vi "Lab Panel V6.00.vi"() -> ()   [LabVIEW 2017] (continued)
                          frame "CHART TEST", Default {
                          }
                          frame "CYCLE TEST" {
                          }
                          frame "T-RISE TEST" {
                          }
                        }
                        n877 = local read "TDMS LAB03-2"() -> (w1509:refnum<k34>)
                        n878 = Build Array("STOPPED") -> (w1506:string[])
                        n879 = Build Array(w1501) -> (w1500:dbl[])
                        n880 = TDMS Write(0:w1509, 5:"TEST RESULT", 7:w1506, 9:w1500) -> (4:w1498:refnum<k34>, 15:w1499:errorcluster)  [unwired: 2 in, 2 out]
                        n881 = TDMS Close(8:w1499, 11:w1498) -> (0:w1497:errorcluster)  [unwired: 1 out]
                      }
                      frame #1 {
                        n882 = local read "DISP LAB03-2"() -> (w1516:T4)
                        n883 = stacked-sequence {
                          tunnel: "LAB03-2" -> [w1518 w1520]
                          frame #0 {
                            n884 = call "sub vi - defrag tdms v1.vi"("panel id"=w1518) -> ("error out"=w1517:errorcluster)  [unwired: 10 in]
                            n885 = local write "data file error"(w1517) -> ()
                          }
                          frame #1 {
                            n886 = call "Save data file (stop) v3.vi"("panel id"=w1520) -> ("network file save error"=w1519:errorcluster)  [unwired: 9 in, 1 out]
                            n887 = local write "RESULT LAB03-2"(FALSE) -> ()
                            n888 = local write "data file error"(w1519) -> ()
                          }
                        }
                        n889 = Bundle(cluster=w1516, "STATUS"="STOP") -> (w1514:T4)  [unwired: 2 in]
                        n890 = local write "DISP LAB03-2"(w1514) -> ()
                      }
                    }
                  }
                  frame True {
                    n891 = local read "SIG LAB03-2"() -> (w1523:T2)
                    n892 = stacked-sequence {
                      seq-local: [w1534 _] -> [_ w1538]
                      tunnel: w1532 -> [_ w1548]
                      tunnel: w1531 -> [_ w1547]
                      tunnel: w1530 -> [_ w1546]
                      tunnel: w1529 -> [_ w1545]
                      tunnel: w1528 -> [_ w1544]
                      tunnel: [_ w1543] -> w1527
                      tunnel: w1526 -> [_ w1542]
                      tunnel: w1525 -> [_ w1541]
                      tunnel: w1524 -> [_ w1540]
                      tunnel: w1523 -> [w1533 w1539]
                      tunnel: w1522 -> [_ w1537]
                      frame #0 {
                        n893 = Unbundle(w1533) -> ("AMPS"=w1536:dbl)  [unwired: 4 out]
                        n894 = call "Check For Amps on v1.vi"("ID"="LAB03-2", "amps"=w1536) -> ("amps"=w1534:bool)  [unwired: 9 in]
                      }
                      frame #1 {
                        n895 = case shown="True" w1538 {
                          tunnel: w1548 -> [_ w1561]
                          tunnel: w1547 -> [_ w1560]
                          tunnel: w1546 -> [_ w1559]
                          tunnel: w1545 -> [_ w1558]
                          tunnel: w1544 -> [_ w1557]
                          tunnel: [errorcluster {"status"=FALSE, "code"=0, "source"=""} ("error out") w1556] -> w1543
                          tunnel: w1542 -> [_ w1555]
                          tunnel: w1541 -> [_ w1554]
                          tunnel: w1540 -> [_ w1553]
                          tunnel: w1539 -> [_ w1552]
                          tunnel: w1537 -> [_ w1551]
                          frame False {
                            w1549 = FALSE
                            n896 = local write "RUN LAB03-2"(w1549) -> ()
                            n897 = local write "run lab03-2"(w1549) -> ()
                          }
                          frame True {
                            n898 = stacked-sequence {
                              seq-local: [w1562 _ _ _ _] -> [_ w1586 _ _ _]
                              tunnel: w1561 -> [w1567 _ _ _ _]
                              tunnel: w1560 -> [w1564 _ _ _ _]
                              tunnel: w1559 -> [w1577 _ _ _ _]
                              tunnel: w1558 -> [w1570 _ _ _ _]
                              tunnel: w1557 -> [w1565 _ _ _ _]
                              tunnel: [_ w1581 _ _ _] -> w1556
                              tunnel: w1555 -> [_ _ _ w1607 _]
                              tunnel: w1554 -> [_ _ _ w1606 _]
                              tunnel: w1553 -> [_ _ _ w1605 _]
                              tunnel: w1552 -> [_ _ _ _ _]
                              tunnel: w1551 -> [_ _ _ _ w1621]
                              frame #0 {
                                w1563 = "\\"
                                n899 = local read "SET LAB03-2"() -> (w1572:T5)
                                n900 = case shown="\"T-RISE TEST\"" w1577 {
                                tunnel: ["L03-2-CHART TEST-" "L03-2-CYCLE TEST-" "L03-2-T-RISE TEST-"] -> w1573
                                frame "CHART TEST", Default {
                                }
                                frame "CYCLE TEST" {
                                }
                                frame "T-RISE TEST" {
                                }
                                }
                                n901 = Unbundle(w1572) -> ("DESCRIPTION"=w1571:string)  [unwired: 4 out]
                                n902 = Concatenate Strings(w1567, "\\", w1565, w1563, w1564, w1563) -> (w1574:string)
                                n903 = String To Path(string=w1574) -> (path=w1576:path)
                                n904 = Concatenate Strings(w1574, w1573, w1571, "-", w1570, ".tdms") -> (w1562:string)
                                n905 = Create Folder(path (use dialog)=w1576) -> (error out=w1575:errorcluster)  [unwired: 2 in, 2 out]
                                n906 = global write "Global 1.vi" "LAB03-2 FILE"(w1562) -> ()
                                n907 = call <vilib>:"Clear Errors.vi"("error in (no error)"=w1575) -> ()  [unwired: 5 in, 2 out]
                              }
                              frame #1 {
                                (unwired) FALSE
                                n908 = String To Path(string=w1586) -> (path=w1582:path)
                                n909 = TDMS Open(6:FALSE, 10:T23."create or replace" ("operation (0:open)"), 11:w1582) -> (0:w1581:errorcluster, 3:→"TDMS LAB03-2":refnum<k34>)  [unwired: 4 in]
                              }
                              frame #2 {
                                n910 = local read "SET LAB03-2"() -> (w1592:T5)
                                n911 = local read "TDMS LAB03-2"() -> (w1603:refnum<k34>)
                                n912 = Build Array("Testers Name", "Description", "Set Test Cycles", "T-Rise minutes", "T-Rise Deg C") -> (w1593:string[])
                                n913 = Unbundle(w1592) -> ("NAME"=w1591:string, "DESCRIPTION"=w1590:string, "CYCLES"=w1589:dbl, "T-RISE mins"=w1588:dbl, "T-RISE deg C"=w1587:dbl)
                                n914 = Number To Decimal String(number=w1589) -> (decimal integer string=w1602:string)  [unwired: 1 in]
                                n915 = Number To Decimal String(number=w1588) -> (decimal integer string=w1601:string)  [unwired: 1 in]
                                n916 = Number To Decimal String(number=w1587) -> (decimal integer string=w1600:string)  [unwired: 1 in]
                                n917 = Build Array(w1591, w1590, w1602, w1601, w1600) -> (w1599:string[])
                                n918 = TDMS Set Properties(5:w1599, 7:w1593, 11:w1603) -> ()  [unwired: 3 in, 4 out]
                              }
                              frame #3 {
                                n919 = local read "DISP LAB03-2"() -> (w1608:T4)
                                n920 = Concatenate Strings("LAB03-2  ", w1607) -> (w1609:string)
                                n921 = Two Button Dialog(message=w1609, 1:w1605, 2:w1606) -> (T button?=w1611:bool)
                                n922 = case shown="True" w1611 {
                                tunnel: w1608 -> [w1618 w1619]
                                tunnel: [w1618 w1619] -> w1615
                                tunnel: [w1617 w1620] -> w1614
                                tunnel: [w1616 w1620] -> w1613
                                frame False {
                                n923 = Unbundle(w1618) -> ("CYCLE"=w1617:dbl, "MINS"=w1616:dbl)  [unwired: 1 out]
                                }
                                frame True {
                                w1620 = 0.0
                                }
                                }
                                n924 = Bundle(cluster=w1615, "CYCLE"=w1614, "MINS"=w1613, "STATUS"="RUN") -> (w1604:T4)
                                n925 = local write "DISP LAB03-2"(w1604) -> ()
                              }
                              frame #4 {
                                n926 = local read "TEMP START LAB03-2"() -> (w1623:cluster{"TL":dbl, "TN":dbl})
                                n927 = Bundle(cluster=w1623, "TL"=w1621, "TN"=w1621) -> (w1622:cluster{"TL":dbl, "TN":dbl})
                                n928 = local write "TEMP START LAB03-2"(w1622) -> ()
                              }
                            }
                          }
                        }
                      }
                    }
                  }
                }
              }
              event "RUN LAB04-1": Value Change {
                n929 = event-data() -> ("NewVal"=w1628:bool)  [unwired: 1 in, 5 out]
                n930 = local write "run lab04-1"(w1628) -> ()
                n931 = case shown="True" w1628 {
                  tunnel: w1634 -> [_ w1672]
                  tunnel: w1633 -> [_ w1671]
                  tunnel: w1631 -> [w1636 w1670]
                  tunnel: w1632 -> [_ w1669]
                  tunnel: w1630 -> [_ w1668]
                  tunnel: [w1635 w1667] -> w1629
                  tunnel: w1627 -> [_ w1666]
                  tunnel: w1626 -> [_ w1665]
                  tunnel: w1625 -> [_ w1664]
                  tunnel: w1624 -> [_ w1662]
                  frame False {
                    # "stop test"
                    n932 = stacked-sequence {
                      tunnel: w1636 -> [w1645 _]
                      tunnel: [w1637 _] -> w1635
                      frame #0 {
                        n933 = local read "DISP LAB04-1"() -> (w1644:T4)
                        n934 = Unbundle(w1644) -> ("CYCLE"=w1642:dbl, "MINS"=w1643:dbl)  [unwired: 1 out]
                        n935 = case shown="\"CYCLE TEST\"" w1645 {
                          tunnel: w1643 -> [_ _ w1652]
                          tunnel: w1642 -> [w1650 w1651 _]
                          tunnel: [w1650 w1651 w1652] -> w1641
                          frame "CHART TEST", Default {
                          }
                          frame "CYCLE TEST" {
                          }
                          frame "T-RISE TEST" {
                          }
                        }
                        n936 = local read "TDMS LAB04-1"() -> (w1649:refnum<k34>)
                        n937 = Build Array("STOPPED") -> (w1646:string[])
                        n938 = Build Array(w1641) -> (w1640:dbl[])
                        n939 = TDMS Write(0:w1649, 5:"TEST RESULT", 7:w1646, 9:w1640) -> (4:w1638:refnum<k34>, 15:w1639:errorcluster)  [unwired: 2 in, 2 out]
                        n940 = TDMS Close(8:w1639, 11:w1638) -> (0:w1637:errorcluster)  [unwired: 1 out]
                      }
                      frame #1 {
                        n941 = local read "DISP LAB04-1"() -> (w1656:T4)
                        n942 = stacked-sequence {
                          tunnel: "LAB04-1" -> [w1658 w1660]
                          frame #0 {
                            n943 = call "sub vi - defrag tdms v1.vi"("panel id"=w1658) -> ("error out"=w1657:errorcluster)  [unwired: 10 in]
                            n944 = local write "data file error"(w1657) -> ()
                          }
                          frame #1 {
                            n945 = call "Save data file (stop) v3.vi"("panel id"=w1660) -> ("network file save error"=w1659:errorcluster)  [unwired: 9 in, 1 out]
                            n946 = local write "RESULT LAB04-1"(FALSE) -> ()
                            n947 = local write "data file error"(w1659) -> ()
                          }
                        }
                        n948 = Bundle(cluster=w1656, "STATUS"="STOP") -> (w1654:T4)  [unwired: 2 in]
                        n949 = local write "DISP LAB04-1"(w1654) -> ()
                      }
                    }
                  }
                  frame True {
                    n950 = local read "SIG LAB04-1"() -> (w1663:T2)
                    n951 = stacked-sequence {
                      seq-local: [w1674 _] -> [_ w1678]
                      tunnel: w1672 -> [_ w1688]
                      tunnel: w1671 -> [_ w1687]
                      tunnel: w1670 -> [_ w1686]
                      tunnel: w1669 -> [_ w1685]
                      tunnel: w1668 -> [_ w1684]
                      tunnel: [_ w1683] -> w1667
                      tunnel: w1666 -> [_ w1682]
                      tunnel: w1665 -> [_ w1681]
                      tunnel: w1664 -> [_ w1680]
                      tunnel: w1663 -> [w1673 w1679]
                      tunnel: w1662 -> [_ w1677]
                      frame #0 {
                        n952 = Unbundle(w1673) -> ("AMPS"=w1676:dbl)  [unwired: 4 out]
                        n953 = call "Check For Amps on v1.vi"("ID"="LAB04-1", "amps"=w1676) -> ("amps"=w1674:bool)  [unwired: 9 in]
                      }
                      frame #1 {
                        n954 = case shown="True" w1678 {
                          tunnel: w1688 -> [_ w1701]
                          tunnel: w1687 -> [_ w1700]
                          tunnel: w1686 -> [_ w1699]
                          tunnel: w1685 -> [_ w1698]
                          tunnel: w1684 -> [_ w1697]
                          tunnel: [errorcluster {"status"=FALSE, "code"=0, "source"=""} ("error out") w1696] -> w1683
                          tunnel: w1682 -> [_ w1695]
                          tunnel: w1681 -> [_ w1694]
                          tunnel: w1680 -> [_ w1693]
                          tunnel: w1679 -> [_ w1692]
                          tunnel: w1677 -> [_ w1691]
                          frame False {
                            w1689 = FALSE
                            n955 = local write "RUN LAB04-1"(w1689) -> ()
                            n956 = local write "run lab04-1"(w1689) -> ()
                          }
                          frame True {
                            n957 = stacked-sequence {
                              seq-local: [w1702 _ _ _ _] -> [_ w1726 _ _ _]
                              tunnel: w1701 -> [w1707 _ _ _ _]
                              tunnel: w1700 -> [w1703 _ _ _ _]
                              tunnel: w1699 -> [w1717 _ _ _ _]
                              tunnel: w1698 -> [w1710 _ _ _ _]
                              tunnel: w1697 -> [w1705 _ _ _ _]
                              tunnel: [_ w1721 _ _ _] -> w1696
                              tunnel: w1695 -> [_ _ _ w1747 _]
                              tunnel: w1694 -> [_ _ _ w1746 _]
                              tunnel: w1693 -> [_ _ _ w1745 _]
                              tunnel: w1692 -> [_ _ _ _ _]
                              tunnel: w1691 -> [_ _ _ _ w1761]
                              frame #0 {
                                w1704 = "\\"
                                n958 = local read "SET LAB04-1"() -> (w1712:T5)
                                n959 = case shown="\"CYCLE TEST\"" w1717 {
                                tunnel: ["L04-1-CHART TEST-" "L04-1-CYCLE TEST-" "L04-1-T-RISE TEST-"] -> w1713
                                frame "CHART TEST", Default {
                                }
                                frame "CYCLE TEST" {
                                }
                                frame "T-RISE TEST" {
                                }
                                }
                                n960 = Unbundle(w1712) -> ("DESCRIPTION"=w1711:string)  [unwired: 4 out]
                                n961 = Concatenate Strings(w1707, "\\", w1705, w1704, w1703, w1704) -> (w1714:string)
                                n962 = String To Path(string=w1714) -> (path=w1716:path)
                                n963 = Concatenate Strings(w1714, w1713, w1711, "-", w1710, ".tdms") -> (w1702:string)
                                n964 = Create Folder(path (use dialog)=w1716) -> (error out=w1715:errorcluster)  [unwired: 2 in, 2 out]
                                n965 = global write "Global 1.vi" "LAB04-1 FILE"(w1702) -> ()
                                n966 = call <vilib>:"Clear Errors.vi"("error in (no error)"=w1715) -> ()  [unwired: 5 in, 2 out]
                              }
                              frame #1 {
                                (unwired) FALSE
                                n967 = String To Path(string=w1726) -> (path=w1722:path)
                                n968 = TDMS Open(6:FALSE, 10:T23."create or replace" ("operation (0:open)"), 11:w1722) -> (0:w1721:errorcluster, 3:→"TDMS LAB04-1":refnum<k34>)  [unwired: 4 in]
                              }
                              frame #2 {
                                n969 = local read "SET LAB04-1"() -> (w1732:T5)
                                n970 = local read "TDMS LAB04-1"() -> (w1743:refnum<k34>)
                                n971 = Build Array("Testers Name", "Description", "Set Test Cycles", "T-Rise minutes", "T-Rise Deg C") -> (w1733:string[])
                                n972 = Unbundle(w1732) -> ("NAME"=w1731:string, "DESCRIPTION"=w1730:string, "CYCLES"=w1729:dbl, "T-RISE mins"=w1728:dbl, "T-RISE deg C"=w1727:dbl)
                                n973 = Number To Decimal String(number=w1729) -> (decimal integer string=w1742:string)  [unwired: 1 in]
                                n974 = Number To Decimal String(number=w1728) -> (decimal integer string=w1741:string)  [unwired: 1 in]
                                n975 = Number To Decimal String(number=w1727) -> (decimal integer string=w1740:string)  [unwired: 1 in]
                                n976 = Build Array(w1731, w1730, w1742, w1741, w1740) -> (w1739:string[])
                                n977 = TDMS Set Properties(5:w1739, 7:w1733, 11:w1743) -> ()  [unwired: 3 in, 4 out]
                              }
                              frame #3 {
                                n978 = local read "DISP LAB04-1"() -> (w1748:T4)
                                n979 = Concatenate Strings("LAB04-1  ", w1747) -> (w1749:string)
                                n980 = Two Button Dialog(message=w1749, 1:w1745, 2:w1746) -> (T button?=w1751:bool)
                                n981 = case shown="True" w1751 {
                                tunnel: w1748 -> [w1758 w1759]
                                tunnel: [w1758 w1759] -> w1755
                                tunnel: [w1757 w1760] -> w1754
                                tunnel: [w1756 w1760] -> w1753
                                frame False {
                                n982 = Unbundle(w1758) -> ("CYCLE"=w1757:dbl, "MINS"=w1756:dbl)  [unwired: 1 out]
                                }
                                frame True {
                                w1760 = 0.0
                                }
                                }
                                n983 = Bundle(cluster=w1755, "CYCLE"=w1754, "MINS"=w1753, "STATUS"="RUN") -> (w1744:T4)
                                n984 = local write "DISP LAB04-1"(w1744) -> ()
                              }
                              frame #4 {
                                n985 = local read "TEMP START LAB04-1"() -> (w1763:cluster{"TL":dbl, "TN":dbl})
                                n986 = Bundle(cluster=w1763, "TL"=w1761, "TN"=w1761) -> (w1762:cluster{"TL":dbl, "TN":dbl})
                                n987 = local write "TEMP START LAB04-1"(w1762) -> ()
                              }
                            }
                          }
                        }
                      }
                    }
                  }
                }
              }
              event "RUN LAB04-2": Value Change {
                n988 = event-data() -> ("NewVal"=w1768:bool)  [unwired: 1 in, 5 out]
                n989 = local write "run lab04-2"(w1768) -> ()
                n990 = case shown="True" w1768 {
                  tunnel: w1774 -> [_ w1812]
                  tunnel: w1773 -> [_ w1811]
                  tunnel: w1771 -> [w1776 w1810]
                  tunnel: w1772 -> [_ w1809]
                  tunnel: w1770 -> [_ w1808]
                  tunnel: [w1775 w1807] -> w1769
                  tunnel: w1767 -> [_ w1806]
                  tunnel: w1766 -> [_ w1805]
                  tunnel: w1765 -> [_ w1804]
                  tunnel: w1764 -> [_ w1802]
                  frame False {
                    # "stop test"
                    n991 = stacked-sequence {
                      tunnel: w1776 -> [w1785 _]
                      tunnel: [w1777 _] -> w1775
                      frame #0 {
                        n992 = local read "DISP LAB04-2"() -> (w1784:T4)
                        n993 = Unbundle(w1784) -> ("CYCLE"=w1782:dbl, "MINS"=w1783:dbl)  [unwired: 1 out]
                        n994 = case shown="\"CYCLE TEST\"" w1785 {
                          tunnel: w1783 -> [_ _ w1792]
                          tunnel: w1782 -> [w1790 w1791 _]
                          tunnel: [w1790 w1791 w1792] -> w1781
                          frame "CHART TEST", Default {
                          }
                          frame "CYCLE TEST" {
                          }
                          frame "T-RISE TEST" {
                          }
                        }
                        n995 = local read "TDMS LAB04-2"() -> (w1789:refnum<k34>)
                        n996 = Build Array("STOPPED") -> (w1786:string[])
                        n997 = Build Array(w1781) -> (w1780:dbl[])
                        n998 = TDMS Write(0:w1789, 5:"TEST RESULT", 7:w1786, 9:w1780) -> (4:w1778:refnum<k34>, 15:w1779:errorcluster)  [unwired: 2 in, 2 out]
                        n999 = TDMS Close(8:w1779, 11:w1778) -> (0:w1777:errorcluster)  [unwired: 1 out]
                      }
                      frame #1 {
                        n1000 = local read "DISP LAB04-2"() -> (w1796:T4)
                        n1001 = stacked-sequence {
                          tunnel: "LAB04-2" -> [w1798 w1800]
                          frame #0 {
                            n1002 = call "sub vi - defrag tdms v1.vi"("panel id"=w1798) -> ("error out"=w1797:errorcluster)  [unwired: 10 in]
                            n1003 = local write "data file error"(w1797) -> ()
                          }
                          frame #1 {
                            n1004 = call "Save data file (stop) v3.vi"("panel id"=w1800) -> ("network file save error"=w1799:errorcluster)  [unwired: 9 in, 1 out]
                            n1005 = local write "RESULT LAB04-2"(FALSE) -> ()
                            n1006 = local write "data file error"(w1799) -> ()
                          }
                        }
                        n1007 = Bundle(cluster=w1796, "STATUS"="STOP") -> (w1794:T4)  [unwired: 2 in]
                        n1008 = local write "DISP LAB04-2"(w1794) -> ()
                      }
                    }
                  }
                  frame True {
                    n1009 = local read "SIG LAB04-2"() -> (w1803:T2)
                    n1010 = stacked-sequence {
                      seq-local: [w1814 _] -> [_ w1818]
                      tunnel: w1812 -> [_ w1828]
                      tunnel: w1811 -> [_ w1827]
                      tunnel: w1810 -> [_ w1826]
                      tunnel: w1809 -> [_ w1825]
                      tunnel: w1808 -> [_ w1824]
                      tunnel: [_ w1823] -> w1807
                      tunnel: w1806 -> [_ w1822]
                      tunnel: w1805 -> [_ w1821]
                      tunnel: w1804 -> [_ w1820]
                      tunnel: w1803 -> [w1813 w1819]
                      tunnel: w1802 -> [_ w1817]
                      frame #0 {
                        n1011 = Unbundle(w1813) -> ("AMPS"=w1816:dbl)  [unwired: 4 out]
                        n1012 = call "Check For Amps on v1.vi"("ID"="LAB04-2", "amps"=w1816) -> ("amps"=w1814:bool)  [unwired: 9 in]
                      }
                      frame #1 {
                        n1013 = case shown="True" w1818 {
                          tunnel: w1828 -> [_ w1841]
                          tunnel: w1827 -> [_ w1840]
                          tunnel: w1826 -> [_ w1839]
                          tunnel: w1825 -> [_ w1838]
                          tunnel: w1824 -> [_ w1837]
                          tunnel: [errorcluster {"status"=FALSE, "code"=0, "source"=""} ("error out") w1836] -> w1823
                          tunnel: w1822 -> [_ w1835]
                          tunnel: w1821 -> [_ w1834]
                          tunnel: w1820 -> [_ w1833]
                          tunnel: w1819 -> [_ w1832]
                          tunnel: w1817 -> [_ w1831]
                          frame False {
                            w1829 = FALSE
                            n1014 = local write "RUN LAB04-2"(w1829) -> ()
                            n1015 = local write "run lab04-2"(w1829) -> ()
                          }
                          frame True {
                            n1016 = stacked-sequence {
                              seq-local: [w1842 _ _ _ _] -> [_ w1866 _ _ _]
                              tunnel: w1841 -> [w1847 _ _ _ _]
                              tunnel: w1840 -> [w1843 _ _ _ _]
                              tunnel: w1839 -> [w1857 _ _ _ _]
                              tunnel: w1838 -> [w1850 _ _ _ _]
                              tunnel: w1837 -> [w1845 _ _ _ _]
                              tunnel: [_ w1861 _ _ _] -> w1836
                              tunnel: w1835 -> [_ _ _ w1887 _]
                              tunnel: w1834 -> [_ _ _ w1886 _]
                              tunnel: w1833 -> [_ _ _ w1885 _]
                              tunnel: w1832 -> [_ _ _ _ _]
                              tunnel: w1831 -> [_ _ _ _ w1901]
                              frame #0 {
                                w1844 = "\\"
                                n1017 = local read "SET LAB04-2"() -> (w1852:T5)
                                n1018 = case shown="\"CHART TEST\", Default" w1857 {
                                tunnel: ["L04-2-CHART TEST-" "L04-2-CYCLE TEST-" "L04-2-T-RISE TEST-"] -> w1853
                                frame "CHART TEST", Default {
                                }
                                frame "CYCLE TEST" {
                                }
                                frame "T-RISE TEST" {
                                }
                                }
                                n1019 = Unbundle(w1852) -> ("DESCRIPTION"=w1851:string)  [unwired: 4 out]
                                n1020 = Concatenate Strings(w1847, "\\", w1845, w1844, w1843, w1844) -> (w1854:string)
                                n1021 = String To Path(string=w1854) -> (path=w1856:path)
                                n1022 = Concatenate Strings(w1854, w1853, w1851, "-", w1850, ".tdms") -> (w1842:string)
                                n1023 = Create Folder(path (use dialog)=w1856) -> (error out=w1855:errorcluster)  [unwired: 2 in, 2 out]
                                n1024 = global write "Global 1.vi" "LAB04-2 FILE"(w1842) -> ()
                                n1025 = call <vilib>:"Clear Errors.vi"("error in (no error)"=w1855) -> ()  [unwired: 5 in, 2 out]
                              }
                              frame #1 {
                                (unwired) FALSE
                                n1026 = String To Path(string=w1866) -> (path=w1862:path)
                                n1027 = TDMS Open(6:FALSE, 10:T23."create or replace" ("operation (0:open)"), 11:w1862) -> (0:w1861:errorcluster, 3:→"TDMS LAB04-2":refnum<k34>)  [unwired: 4 in]
                              }
                              frame #2 {
                                n1028 = local read "SET LAB04-2"() -> (w1872:T5)
                                n1029 = local read "TDMS LAB04-2"() -> (w1883:refnum<k34>)
                                n1030 = Build Array("Testers Name", "Description", "Set Test Cycles", "T-Rise minutes", "T-Rise Deg C") -> (w1873:string[])
                                n1031 = Unbundle(w1872) -> ("NAME"=w1871:string, "DESCRIPTION"=w1870:string, "CYCLES"=w1869:dbl, "T-RISE mins"=w1868:dbl, "T-RISE deg C"=w1867:dbl)
                                n1032 = Number To Decimal String(number=w1869) -> (decimal integer string=w1882:string)  [unwired: 1 in]
                                n1033 = Number To Decimal String(number=w1868) -> (decimal integer string=w1881:string)  [unwired: 1 in]
                                n1034 = Number To Decimal String(number=w1867) -> (decimal integer string=w1880:string)  [unwired: 1 in]
                                n1035 = Build Array(w1871, w1870, w1882, w1881, w1880) -> (w1879:string[])
                                n1036 = TDMS Set Properties(5:w1879, 7:w1873, 11:w1883) -> ()  [unwired: 3 in, 4 out]
                              }
                              frame #3 {
                                n1037 = local read "DISP LAB04-2"() -> (w1888:T4)
                                n1038 = Concatenate Strings("LAB04-2 ", w1887) -> (w1889:string)
                                n1039 = Two Button Dialog(message=w1889, 1:w1885, 2:w1886) -> (T button?=w1891:bool)
                                n1040 = case shown="True" w1891 {
                                tunnel: w1888 -> [w1898 w1899]
                                tunnel: [w1898 w1899] -> w1895
                                tunnel: [w1897 w1900] -> w1894
                                tunnel: [w1896 w1900] -> w1893
                                frame False {
                                n1041 = Unbundle(w1898) -> ("CYCLE"=w1897:dbl, "MINS"=w1896:dbl)  [unwired: 1 out]
                                }
                                frame True {
                                w1900 = 0.0
                                }
                                }
                                n1042 = Bundle(cluster=w1895, "CYCLE"=w1894, "MINS"=w1893, "STATUS"="RUN") -> (w1884:T4)
                                n1043 = local write "DISP LAB04-2"(w1884) -> ()
                              }
                              frame #4 {
                                n1044 = local read "TEMP START LAB04-2"() -> (w1903:cluster{"TL":dbl, "TN":dbl})
                                n1045 = Bundle(cluster=w1903, "TL"=w1901, "TN"=w1901) -> (w1902:cluster{"TL":dbl, "TN":dbl})
                                n1046 = local write "TEMP START LAB04-2"(w1902) -> ()
                              }
                            }
                          }
                        }
                      }
                    }
                  }
                }
              }
              event "RUN LAB05-1": Value Change {
                n1047 = event-data() -> ("NewVal"=w1908:bool)  [unwired: 1 in, 5 out]
                n1048 = local write "run lab05-1"(w1908) -> ()
                n1049 = case shown="True" w1908 {
                  tunnel: w1914 -> [_ w1952]
                  tunnel: w1913 -> [_ w1951]
                  tunnel: w1911 -> [w1916 w1950]
                  tunnel: w1912 -> [_ w1949]
                  tunnel: w1910 -> [_ w1948]
                  tunnel: [w1915 w1947] -> w1909
                  tunnel: w1907 -> [_ w1946]
                  tunnel: w1906 -> [_ w1945]
                  tunnel: w1905 -> [_ w1944]
                  tunnel: w1904 -> [_ w1942]
                  frame False {
                    # "stop test"
                    n1050 = stacked-sequence {
                      tunnel: w1916 -> [w1925 _]
                      tunnel: [w1917 _] -> w1915
                      frame #0 {
                        n1051 = local read "DISP LAB05-1"() -> (w1924:T4)
                        n1052 = Unbundle(w1924) -> ("CYCLE"=w1922:dbl, "MINS"=w1923:dbl)  [unwired: 1 out]
                        n1053 = case shown="\"CYCLE TEST\"" w1925 {
                          tunnel: w1923 -> [_ _ w1932]
                          tunnel: w1922 -> [w1930 w1931 _]
                          tunnel: [w1930 w1931 w1932] -> w1921
                          frame "CHART TEST", Default {
                          }
                          frame "CYCLE TEST" {
                          }
                          frame "T-RISE TEST" {
                          }
                        }
                        n1054 = local read "TDMS LAB05-1"() -> (w1929:refnum<k34>)
                        n1055 = Build Array("STOPPED") -> (w1926:string[])
                        n1056 = Build Array(w1921) -> (w1920:dbl[])
                        n1057 = TDMS Write(0:w1929, 5:"TEST RESULT", 7:w1926, 9:w1920) -> (4:w1918:refnum<k34>, 15:w1919:errorcluster)  [unwired: 2 in, 2 out]
                        n1058 = TDMS Close(8:w1919, 11:w1918) -> (0:w1917:errorcluster)  [unwired: 1 out]
                      }
                      frame #1 {
                        n1059 = local read "DISP LAB05-1"() -> (w1936:T4)
                        n1060 = stacked-sequence {
                          tunnel: "LAB05-1" -> [w1938 w1940]
                          frame #0 {
                            n1061 = call "sub vi - defrag tdms v1.vi"("panel id"=w1938) -> ("error out"=w1937:errorcluster)  [unwired: 10 in]
                            n1062 = local write "data file error"(w1937) -> ()
                          }
                          frame #1 {
                            n1063 = call "Save data file (stop) v3.vi"("panel id"=w1940) -> ("network file save error"=w1939:errorcluster)  [unwired: 9 in, 1 out]
                            n1064 = local write "RESULT LAB05-1"(FALSE) -> ()
                            n1065 = local write "data file error"(w1939) -> ()
                          }
                        }
                        n1066 = Bundle(cluster=w1936, "STATUS"="STOP") -> (w1934:T4)  [unwired: 2 in]
                        n1067 = local write "DISP LAB05-1"(w1934) -> ()
                      }
                    }
                  }
                  frame True {
                    n1068 = local read "SIG LAB05-1"() -> (w1943:T2)
                    n1069 = stacked-sequence {
                      seq-local: [w1954 _] -> [_ w1958]
                      tunnel: w1952 -> [_ w1968]
                      tunnel: w1951 -> [_ w1967]
                      tunnel: w1950 -> [_ w1966]
                      tunnel: w1949 -> [_ w1965]
                      tunnel: w1948 -> [_ w1964]
                      tunnel: [_ w1963] -> w1947
                      tunnel: w1946 -> [_ w1962]
                      tunnel: w1945 -> [_ w1961]
                      tunnel: w1944 -> [_ w1960]
                      tunnel: w1943 -> [w1953 w1959]
                      tunnel: w1942 -> [_ w1957]
                      frame #0 {
                        n1070 = Unbundle(w1953) -> ("AMPS"=w1956:dbl)  [unwired: 4 out]
                        n1071 = call "Check For Amps on v1.vi"("ID"="LAB05-1", "amps"=w1956) -> ("amps"=w1954:bool)  [unwired: 9 in]
                      }
                      frame #1 {
                        n1072 = case shown="True" w1958 {
                          tunnel: w1968 -> [_ w1981]
                          tunnel: w1967 -> [_ w1980]
                          tunnel: w1966 -> [_ w1979]
                          tunnel: w1965 -> [_ w1978]
                          tunnel: w1964 -> [_ w1977]
                          tunnel: [errorcluster {"status"=FALSE, "code"=0, "source"=""} ("error out") w1976] -> w1963
                          tunnel: w1962 -> [_ w1975]
                          tunnel: w1961 -> [_ w1974]
                          tunnel: w1960 -> [_ w1973]
                          tunnel: w1959 -> [_ w1972]
                          tunnel: w1957 -> [_ w1971]
                          frame False {
                            w1969 = FALSE
                            n1073 = local write "RUN LAB05-1"(w1969) -> ()
                            n1074 = local write "run lab05-1"(w1969) -> ()
                          }
                          frame True {
                            n1075 = stacked-sequence {
                              seq-local: [w1982 _ _ _ _] -> [_ w2006 _ _ _]
                              tunnel: w1981 -> [w1987 _ _ _ _]
                              tunnel: w1980 -> [w1983 _ _ _ _]
                              tunnel: w1979 -> [w1997 _ _ _ _]
                              tunnel: w1978 -> [w1990 _ _ _ _]
                              tunnel: w1977 -> [w1985 _ _ _ _]
                              tunnel: [_ w2001 _ _ _] -> w1976
                              tunnel: w1975 -> [_ _ _ w2026 _]
                              tunnel: w1974 -> [_ _ _ w2025 _]
                              tunnel: w1973 -> [_ _ _ w2024 _]
                              tunnel: w1972 -> [_ _ _ _ _]
                              tunnel: w1971 -> [_ _ _ _ w2041]
                              frame #0 {
                                w1984 = "\\"
                                n1076 = local read "SET LAB05-1"() -> (w1992:T5)
                                n1077 = case shown="\"CYCLE TEST\"" w1997 {
                                tunnel: ["L05-1-CHART TEST-" "L05-1-CYCLE TEST-" "L05-1-T-RISE TEST-"] -> w1993
                                frame "CHART TEST", Default {
                                }
                                frame "CYCLE TEST" {
                                }
                                frame "T-RISE TEST" {
                                }
                                }
                                n1078 = Unbundle(w1992) -> ("DESCRIPTION"=w1991:string)  [unwired: 4 out]
                                n1079 = Concatenate Strings(w1987, "\\", w1985, w1984, w1983, w1984) -> (w1994:string)
                                n1080 = String To Path(string=w1994) -> (path=w1996:path)
                                n1081 = Concatenate Strings(w1994, w1993, w1991, "-", w1990, ".tdms") -> (w1982:string)
                                n1082 = Create Folder(path (use dialog)=w1996) -> (error out=w1995:errorcluster)  [unwired: 2 in, 2 out]
                                n1083 = global write "Global 1.vi" "LAB05-1 FILE"(w1982) -> ()
                                n1084 = call <vilib>:"Clear Errors.vi"("error in (no error)"=w1995) -> ()  [unwired: 5 in, 2 out]
                              }
                              frame #1 {
                                (unwired) FALSE
                                n1085 = String To Path(string=w2006) -> (path=w2002:path)
                                n1086 = TDMS Open(6:FALSE, 10:T23."create or replace" ("operation (0:open)"), 11:w2002) -> (0:w2001:errorcluster, 3:→"TDMS LAB05-1":refnum<k34>)  [unwired: 4 in]
                              }
                              frame #2 {
                                n1087 = local read "SET LAB05-1"() -> (w2012:T5)
                                n1088 = local read "TDMS LAB05-1"() -> (w2023:refnum<k34>)
                                n1089 = Build Array("Testers Name", "Description", "Set Test Cycles", "T-Rise minutes", "T-Rise Deg C") -> (w2013:string[])
                                n1090 = Unbundle(w2012) -> ("NAME"=w2011:string, "DESCRIPTION"=w2010:string, "CYCLES"=w2009:dbl, "T-RISE mins"=w2008:dbl, "T-RISE deg C"=w2007:dbl)
                                n1091 = Number To Decimal String(number=w2009) -> (decimal integer string=w2022:string)  [unwired: 1 in]
                                n1092 = Number To Decimal String(number=w2008) -> (decimal integer string=w2021:string)  [unwired: 1 in]
                                n1093 = Number To Decimal String(number=w2007) -> (decimal integer string=w2020:string)  [unwired: 1 in]
                                n1094 = Build Array(w2011, w2010, w2022, w2021, w2020) -> (w2019:string[])
                                n1095 = TDMS Set Properties(5:w2019, 7:w2013, 11:w2023) -> ()  [unwired: 3 in, 4 out]
                              }
                              frame #3 {
                                n1096 = local read "DISP LAB05-1"() -> (w2028:T4)
                                n1097 = Concatenate Strings("LAB05-1  ", w2026) -> (w2029:string)
                                n1098 = Two Button Dialog(message=w2029, 1:w2024, 2:w2025) -> (T button?=w2031:bool)
                                n1099 = case shown="True" w2031 {
                                tunnel: w2028 -> [w2038 w2039]
                                tunnel: [w2038 w2039] -> w2035
                                tunnel: [w2037 w2040] -> w2034
                                tunnel: [w2036 w2040] -> w2033
                                frame False {
                                n1100 = Unbundle(w2038) -> ("CYCLE"=w2037:dbl, "MINS"=w2036:dbl)  [unwired: 1 out]
                                }
                                frame True {
                                w2040 = 0.0
                                }
                                }
                                n1101 = Bundle(cluster=w2035, "CYCLE"=w2034, "MINS"=w2033, "STATUS"="RUN") -> (w2027:T4)
                                n1102 = local write "DISP LAB05-1"(w2027) -> ()
                              }
                              frame #4 {
                                n1103 = local read "TEMP START LAB05-1"() -> (w2043:cluster{"TL":dbl, "TN":dbl})
                                n1104 = Bundle(cluster=w2043, "TL"=w2041, "TN"=w2041) -> (w2042:cluster{"TL":dbl, "TN":dbl})
                                n1105 = local write "TEMP START LAB05-1"(w2042) -> ()
                              }
                            }
                          }
                        }
                      }
                    }
                  }
                }
              }
              event "RUN LAB05-2": Value Change {
                n1106 = event-data() -> ("NewVal"=w2049:bool)  [unwired: 1 in, 5 out]
                n1107 = local read "SIG LAB05-2"() -> (w2045:T2)
                n1108 = case shown="True" w2049 {
                  tunnel: w2055 -> [_ w2093]
                  tunnel: w2054 -> [_ w2092]
                  tunnel: w2052 -> [w2057 w2091]
                  tunnel: w2053 -> [_ w2090]
                  tunnel: w2051 -> [_ w2089]
                  tunnel: [w2056 w2088] -> w2050
                  tunnel: w2048 -> [_ w2087]
                  tunnel: w2047 -> [_ w2086]
                  tunnel: w2046 -> [_ w2085]
                  tunnel: w2045 -> [_ w2084]
                  tunnel: w2044 -> [_ w2083]
                  frame False {
                    # "stop test"
                    n1109 = stacked-sequence {
                      tunnel: w2057 -> [w2066 _]
                      tunnel: [w2058 _] -> w2056
                      frame #0 {
                        n1110 = local read "DISP LAB05-2"() -> (w2065:T4)
                        n1111 = Unbundle(w2065) -> ("CYCLE"=w2063:dbl, "MINS"=w2064:dbl)  [unwired: 1 out]
                        n1112 = case shown="\"CYCLE TEST\"" w2066 {
                          tunnel: w2064 -> [_ _ w2073]
                          tunnel: w2063 -> [w2071 w2072 _]
                          tunnel: [w2071 w2072 w2073] -> w2062
                          frame "CHART TEST", Default {
                          }
                          frame "CYCLE TEST" {
                          }
                          frame "T-RISE TEST" {
                          }
                        }
                        n1113 = local read "TDMS LAB05-2"() -> (w2070:refnum<k34>)
                        n1114 = Build Array("STOPPED") -> (w2067:string[])
                        n1115 = Build Array(w2062) -> (w2061:dbl[])
                        n1116 = TDMS Write(0:w2070, 5:"TEST RESULT", 7:w2067, 9:w2061) -> (4:w2059:refnum<k34>, 15:w2060:errorcluster)  [unwired: 2 in, 2 out]
                        n1117 = TDMS Close(8:w2060, 11:w2059) -> (0:w2058:errorcluster)  [unwired: 1 out]
                      }
                      frame #1 {
                        n1118 = local read "DISP LAB05-2"() -> (w2077:T4)
                        n1119 = stacked-sequence {
                          tunnel: "LAB05-2" -> [w2079 w2081]
                          frame #0 {
                            n1120 = call "sub vi - defrag tdms v1.vi"("panel id"=w2079) -> ("error out"=w2078:errorcluster)  [unwired: 10 in]
                            n1121 = local write "data file error"(w2078) -> ()
                          }
                          frame #1 {
                            n1122 = local write "RESULT LAB05-2"(FALSE) -> ()
                            n1123 = call "Save data file (stop) v3.vi"("panel id"=w2081) -> ("network file save error"=w2080:errorcluster)  [unwired: 9 in, 1 out]
                            n1124 = local write "data file error"(w2080) -> ()
                          }
                        }
                        n1125 = Bundle(cluster=w2077, "STATUS"="STOP") -> (w2075:T4)  [unwired: 2 in]
                        n1126 = local write "DISP LAB05-2"(w2075) -> ()
                      }
                    }
                  }
                  frame True {
                    n1127 = stacked-sequence {
                      seq-local: [w2095 _] -> [_ w2099]
                      tunnel: w2093 -> [_ w2109]
                      tunnel: w2092 -> [_ w2108]
                      tunnel: w2091 -> [_ w2107]
                      tunnel: w2090 -> [_ w2106]
                      tunnel: w2089 -> [_ w2105]
                      tunnel: [_ w2104] -> w2088
                      tunnel: w2087 -> [_ w2103]
                      tunnel: w2086 -> [_ w2102]
                      tunnel: w2085 -> [_ w2101]
                      tunnel: w2084 -> [w2094 w2100]
                      tunnel: w2083 -> [_ w2098]
                      frame #0 {
                        n1128 = Unbundle(w2094) -> ("AMPS"=w2097:dbl)  [unwired: 4 out]
                        n1129 = call "Check For Amps on v1.vi"("ID"="LAB05-2", "amps"=w2097) -> ("amps"=w2095:bool)  [unwired: 9 in]
                      }
                      frame #1 {
                        n1130 = case shown="True" w2099 {
                          tunnel: w2109 -> [_ w2121]
                          tunnel: w2108 -> [_ w2119]
                          tunnel: w2107 -> [_ w2116]
                          tunnel: w2106 -> [_ w2117]
                          tunnel: w2105 -> [_ w2120]
                          tunnel: [errorcluster {"status"=FALSE, "code"=0, "source"=""} ("error out") w2112] -> w2104
                          tunnel: w2103 -> [_ w2115]
                          tunnel: w2102 -> [_ w2114]
                          tunnel: w2101 -> [_ w2113]
                          tunnel: w2100 -> [_ w2118]
                          tunnel: w2098 -> [_ w2122]
                          frame False {
                            w2110 = FALSE
                            n1131 = local write "RUN LAB05-2"(w2110) -> ()
                            n1132 = local write "run lab05-2"(w2110) -> ()
                          }
                          frame True {
                            n1133 = stacked-sequence {
                              seq-local: [w2123 _ _ _ _] -> [_ w2147 _ _ _]
                              tunnel: w2121 -> [w2128 _ _ _ _]
                              tunnel: w2119 -> [w2124 _ _ _ _]
                              tunnel: w2116 -> [w2138 _ _ _ _]
                              tunnel: w2117 -> [w2131 _ _ _ _]
                              tunnel: w2120 -> [w2126 _ _ _ _]
                              tunnel: [_ w2142 _ _ _] -> w2112
                              tunnel: w2115 -> [_ _ _ w2167 _]
                              tunnel: w2114 -> [_ _ _ w2166 _]
                              tunnel: w2113 -> [_ _ _ w2165 _]
                              tunnel: w2118 -> [_ _ _ _ _]
                              tunnel: w2122 -> [_ _ _ _ w2182]
                              frame #0 {
                                w2125 = "\\"
                                n1134 = local read "SET LAB05-2"() -> (w2133:T5)
                                n1135 = case shown="\"CYCLE TEST\"" w2138 {
                                tunnel: ["L05-2-CHART TEST-" "L05-2-CYCLE TEST-" "L05-2-T-RISE TEST-"] -> w2134
                                frame "CHART TEST", Default {
                                }
                                frame "CYCLE TEST" {
                                }
                                frame "T-RISE TEST" {
                                }
                                }
                                n1136 = Unbundle(w2133) -> ("DESCRIPTION"=w2132:string)  [unwired: 4 out]
                                n1137 = Concatenate Strings(w2128, "\\", w2126, w2125, w2124, w2125) -> (w2135:string)
                                n1138 = String To Path(string=w2135) -> (path=w2137:path)
                                n1139 = Concatenate Strings(w2135, w2134, w2132, "-", w2131, ".tdms") -> (w2123:string)
                                n1140 = Create Folder(path (use dialog)=w2137) -> (error out=w2136:errorcluster)  [unwired: 2 in, 2 out]
                                n1141 = global write "Global 1.vi" "LAB05-2 FILE"(w2123) -> ()
                                n1142 = call <vilib>:"Clear Errors.vi"("error in (no error)"=w2136) -> ()  [unwired: 5 in, 2 out]
                              }
                              frame #1 {
                                (unwired) FALSE
                                n1143 = String To Path(string=w2147) -> (path=w2143:path)
